vi "CLD 11 CSV file utility.vi"(8 "Error In":errorcluster, 10 "[Data In]":T1[](array[typedef]), 11 "CSV File Enum":T2) -> (0 "Error Out":errorcluster, 3 "[Data Out]":T1[](array[typedef]))   [LabVIEW 2018]
doc: "CLD 11 File utility from CLD 6"
uses:
  CLD 11 CSV file enum.ctl
  CLD 11 CSV file data structure.ctl
  <vilib>/Utility/file.llb/Read Delimited Spreadsheet (string).vi
  <vilib>/Utility/file.llb/Write To Spreadsheet File (string).vi
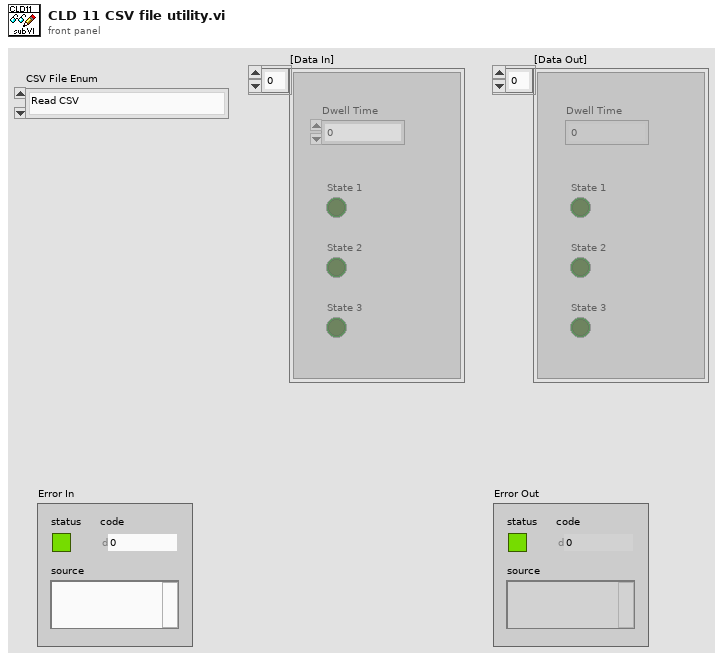
[diagram p1: front panel]
types:
  T1 = typedef "CLD 11 CSV file data structure.ctl" = cluster{"Dwell Time":i32, "State 1":bool, "State 2":bool, "State 3":bool}
  T2 = typedef "CLD 11 CSV file enum.ctl" = enum16{"Read CSV", "Write CSV"}
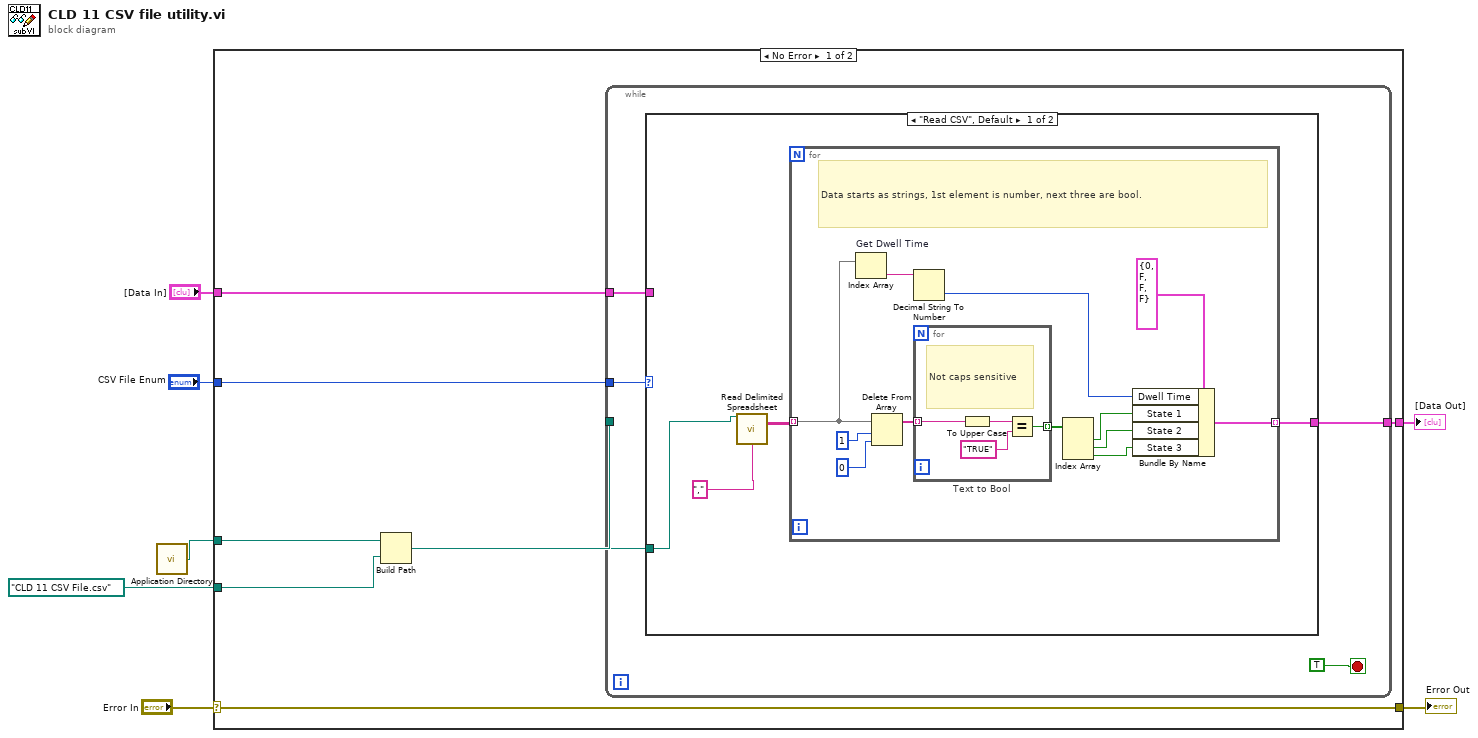
[diagram p0: block diagram]
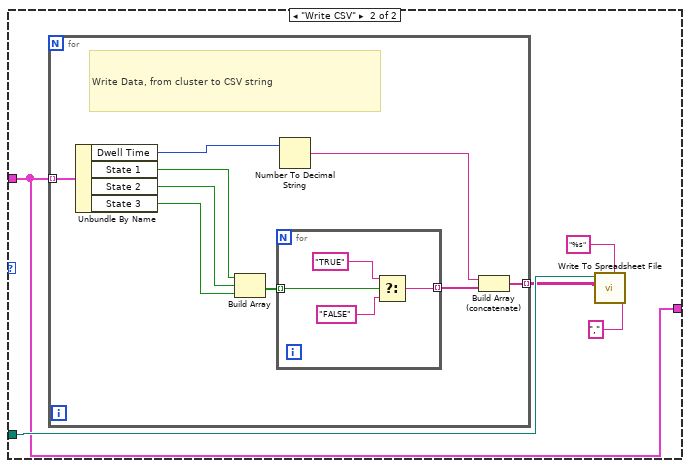
[diagram p2: hidden frame]
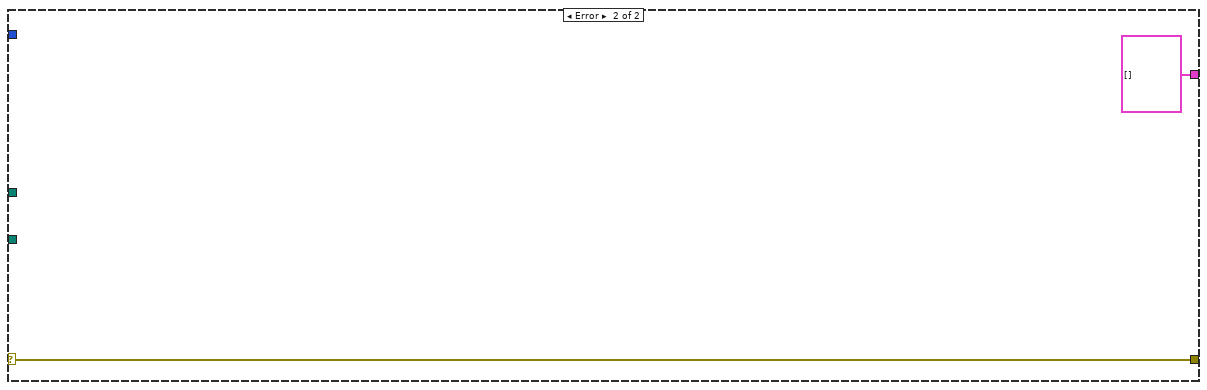
[diagram p3: hidden frame]
diagram:
  n1 = call <vilib>:"Application Directory.vi"() -> ("Application Directory"=w1:path)
  n2 = case shown="No Error" "Error In" {
    selector: "Error In" -> [w9 w59]
    tunnel: [w14 T1[] [] ("[Data In]")] -> w7
    tunnel: path "CLD 11 CSV File.csv" -> [w13 _]
    tunnel: "CSV File Enum" -> [w11 _]
    tunnel: "[Data In]" -> [w10 _]
    tunnel: [w9 w59] -> w2
    tunnel: w1 -> [w8 _]
    frame No Error {
      n3 = Build Path(base path=w8, name or relative path=w13) -> (appended path=w12:path)
      n4 = while {
        tunnel: w12 -> [w17]
        tunnel: w11 -> [w18]
        tunnel: [w16] -> w14
        tunnel: w10 -> [w15]
        stop <- TRUE stop-if-true
        n5 = case shown="\"Read CSV\", Default" w18 {
          tunnel: w17 -> [w22 w44]
          tunnel: [w23 w40] -> w16
          tunnel: w15 -> [_ w40]
          frame "Read CSV", Default {
            n6 = call-poly <vilib>:"Read Delimited Spreadsheet.vi"("file path (dialog if empty)"=w22, "delimiter (\\t)"="," ("delimiter (\\t)")) -> ("all rows"=w21:string[][])  [unwired: 8 in, 5 out]
            n7 = for {
              tunnel: w21 -> [w32] mode=indexing
              tunnel: [w35] -> w23 mode=indexing
              # "Data starts as strings, 1st element is number, next three are bool."
              n8 = Index Array "Get Dwell Time"(array=w32) -> (element=w34:string)  [unwired: 1 in]
              n9 = Delete From Array(array=w32, length=1, index=0) -> (array with subset deleted=w25:string[])  [unwired: 1 out]
              n10 = Decimal String To Number(string=w34) -> (number=w33:i32)  [unwired: 2 in, 1 out]
              n11 = for "Text to Bool" {
                tunnel: w25 -> [w39] mode=indexing
                tunnel: [w36] -> w29 mode=indexing
                # "Not caps sensitive"
                n12 = To Upper Case(1:w39) -> (0:w38:string)
                n13 = Equal?(x=w38, y="TRUE") -> (x = y?=w36:bool)
              }
              n14 = Index Array(array=w29) -> (element #1=w28:bool, element #2=w27:bool, element #3=w26:bool)  [unwired: 3 in]
              n15 = Bundle By Name(cluster=T1 {"Dwell Time"=0, "State 1"=FALSE, "State 2"=FALSE, "State 3"=FALSE} ("CSV File Data Structure"), "Dwell Time"=w33, "State 1"=w28, "State 2"=w27, "State 3"=w26) -> (w35:T1)
            }
          }
          frame "Write CSV" {
            n16 = for {
              tunnel: w40 -> [w53] mode=indexing
              tunnel: [w45] -> w42 mode=indexing
              # "Write Data, from cluster to CSV string"
              n17 = Unbundle By Name(w53) -> ("Dwell Time"=w52:i32, "State 1"=w51:bool, "State 2"=w50:bool, "State 3"=w49:bool)
              n18 = Build Array(w51, w50, w49) -> (w48:bool[])
              n19 = for {
                tunnel: w48 -> [w57] mode=indexing
                tunnel: [w54] -> w46 mode=indexing
                n20 = Select(t="TRUE", s=w57, f="FALSE") -> (s? t:f=w54:string)
              }
              n21 = Number To Decimal String(number=w52) -> (decimal integer string=w47:string)  [unwired: 1 in]
              n22 = Build Array (concatenate)(w47, w46) -> (w45:string[])
            }
            n23 = call-poly <vilib>:"Write To Spreadsheet File.vi"("delimiter (\\t)"="," ("delimiter (\\t)"), "format (%s)"="%s", "2D data"=w42, "file path (dialog if empty)"=w44) -> ()  [unwired: 4 in, 1 out]
          }
        }
      }
    }
    frame Error {
    }
  }
  "[Data Out]" <- w7
  "Error Out" <- w2
